vi "Handle Pos and Rot.vi"(5 "Mouse Up":bool, 6 "Delta":bool, 7 "Picture in":refnum<vi>, 8 "Option":T1, 9 "Coord (ft)":cluster{dbl, dbl}, 10 "Index":i32, 11 "Points in":cluster{"x":dbl, "y":dbl, "th":dbl}[](array[cluster])) -> (3 "Points out":cluster{"x":dbl, "y":dbl, "th":dbl}[](array[cluster]))   [LabVIEW 2019]
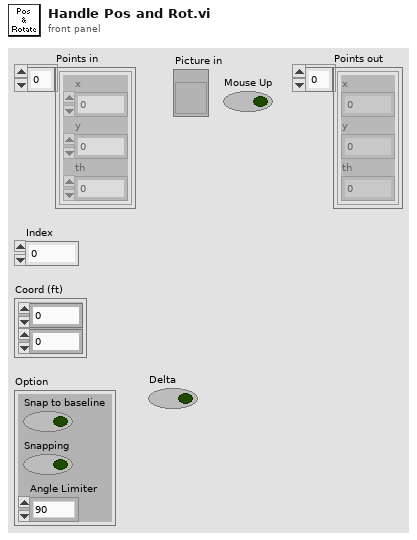
[diagram p1: front panel]
types:
  T1 = cluster{"Snap to baseline":bool, "Snapping":bool, "Angle Limiter":enum16{"90", "45", "15", "1"}}
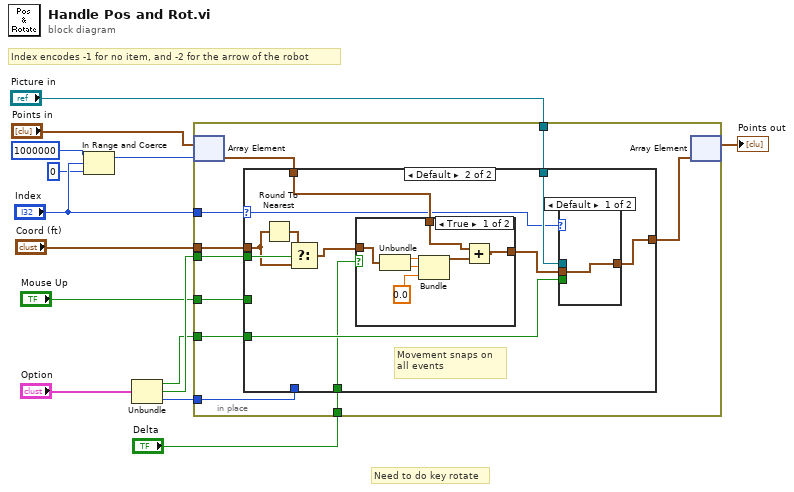
[diagram p0: block diagram]
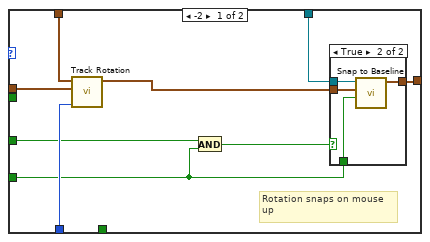
[diagram p2: hidden frame]
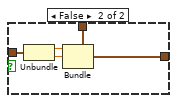
[diagram p4: hidden frame]
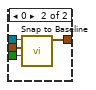
[diagram p5: hidden frame]
diagram:
  # "Need to do key rotate"
  # "Index encodes -1 for no item, and -2 for the arrow of the robot"
  n1 = In Range and Coerce(upper limit=1000000 ("lower limit"), x="Index", lower limit=0) -> (coerced(x)=w2:i32)  [unwired: 1 out]
  n2 = Unbundle("Option") -> ("Snap to baseline"=w12:bool, "Snapping"=w13:bool, "Angle Limiter"=w14:enum16{"90", "45", "15", "1"})
  n3 = in-place {
    in-place-border: "Coord (ft)" -> [w24]
    in-place-border: "Index" -> [w21]
    in-place-border: w13 -> [w20]
    in-place-border: w12 -> [w18]
    in-place-border: w14 -> [w19]
    in-place-border: "Picture in" -> [w17]
    in-place-border: "Mouse Up" -> [w16]
    in-place-border: "Delta" -> [w15]
    n4 = in-place-array #1("Points in", w2) -> (w23:cluster{"x":dbl, "y":dbl, "th":dbl})
    n5 = case shown="Default" w21 {
      selector: w21 -> [_ w40]
      tunnel: w24 -> [w33 w47]
      tunnel: w23 -> [w25 w42]
      tunnel: [w26 w41] -> w22
      tunnel: w19 -> [w32 _]
      tunnel: w20 -> [_ w49]
      tunnel: w18 -> [w28 w45]
      tunnel: w17 -> [w31 w43]
      tunnel: w16 -> [w30 _]
      tunnel: w15 -> [_ w39]
      frame -2 {
        # "Rotation snaps on mouse\nup"
        n6 = call "Track Rotation.vi"("Angle Limiter"=w32, "Coord"=w33, "Point in"=w25) -> ("Point out"=w27:cluster{"x":dbl, "y":dbl, "th":dbl})  [unwired: 8 in]
        n7 = And(x=w30, y=w28) -> (x .and. y?=w29:bool)
        n8 = case shown="True" w29 {
          tunnel: w27 -> [w34 w36]
          tunnel: [w34 w38] -> w26
          tunnel: w31 -> [_ w37]
          tunnel: w28 -> [_ w35]
          frame False {
          }
          frame True {
            n9 = call "Snap to Baseline.vi"("Snap to baseline"=w35, "Point in"=w36, "Picture in"=w37) -> ("Point out"=w38:cluster{"x":dbl, "y":dbl, "th":dbl})  [unwired: 8 in]
          }
        }
      }
      frame Default {
        # "Movement snaps on\nall events"
        n10 = Round To Nearest(number=w47) -> (nearest integer value=w48:cluster{dbl, dbl})
        n11 = Select(t=w48, s=w49, f=w47) -> (s? t:f=w46:cluster{dbl, dbl})
        n12 = case shown="True" w39 {
          tunnel: w46 -> [w56 w59]
          tunnel: [w52 w58] -> w44
          tunnel: w42 -> [w50 w57]
          frame True {
            n13 = Unbundle(w56) -> (w55:dbl, w54:dbl)
            n14 = Bundle(w55, w54, 0.0) -> (w51:cluster{dbl, dbl, dbl})  [unwired: 1 in]
            n15 = Add(x=w50, y=w51) -> (x+y=w52:cluster{dbl, dbl, dbl})
          }
          frame False {
            n16 = Unbundle(w59) -> (w61:dbl, w60:dbl)
            n17 = Bundle(cluster=w57, "x"=w61, "y"=w60) -> (w58:cluster{"x":dbl, "y":dbl, "th":dbl})  [unwired: 1 in]
          }
        }
        n18 = case shown="Default" w40 {
          tunnel: w45 -> [_ w66]
          tunnel: w44 -> [w62 w65]
          tunnel: w43 -> [_ w64]
          tunnel: [w62 w63] -> w41
          frame Default {
          }
          frame 0 {
            n19 = call "Snap to Baseline.vi"("Snap to baseline"=w66, "Point in"=w65, "Picture in"=w64) -> ("Point out"=w63:cluster{"x":dbl, "y":dbl, "th":dbl})  [unwired: 8 in]
          }
        }
      }
    }
    n20 = in-place-array #1(w22) -> (→"Points out":cluster{"x":dbl, "y":dbl, "th":dbl}[])  [unwired: 1 out]
  }
